vi "zmq_has.vi"(3 "error in":errorcluster, 5 "capabilty":string(combo)) -> (0 "error out":errorcluster, 2 "provided":bool)   [LabVIEW 2025, in "ZeroMQ.lvlib"]
doc: "Checks whether a particular functionality was compiled into the ZMQ library\n\nDetailed API documentation: http://api.zeromq.org/master:zmq-has"
uses:
  ZeroMQ.lvlib
panel:
  # "ØMQ"
  # "labview"
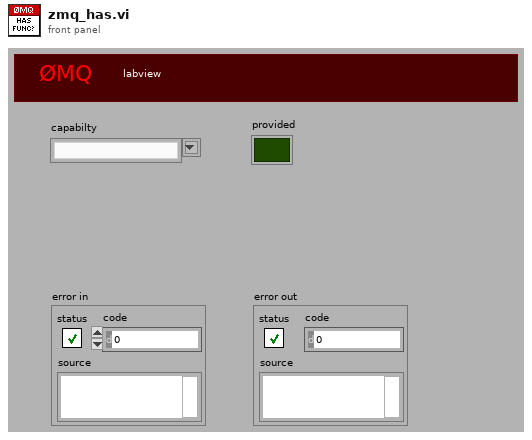
[diagram p1: front panel]
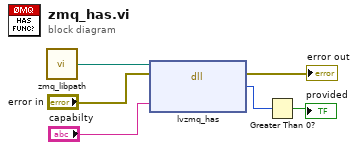
[diagram p0: block diagram]
diagram:
  n1 = call "zmq_libpath.vi"() -> ("path"=w6:path)
  n2 = dll-call lib="?" fn="lvzmq_has" ("zmq_labview.dll:lvzmq_socket")(path in=w6, error in="error in", "capability"="capabilty") -> (error out=→"error out":errorcluster, "return type"=w4:i32)  [unwired: 2 in, 1 out]
  n3 = Greater Than 0?(x=w4) -> (x > 0?=→"provided":bool)
